vi "PruebaCalibration.vi"() -> ()   [LabVIEW 2014, in "MSX-E3701_dll.lvlib"]
uses:
  MSX-E3701_dll.lvlib
  E:/Repositorio Magnis/INF002/v0/Modules/HAL/Drivers/Sync/ADDI-DATA MSX-E3701/API/MX370x.dll
  MX370x.dll
  Typedef/Connection Data.ctl
  E:/Repositorio Magnis/INF002/v0/Modules/HAL/Drivers/Sync/ADDI-DATA MSX-E3701/API/MXCommon.dll
  MXCommon.dll
panel:
  in  "Connection Data In":T1
  out "ulValue":u64
  out "TransducerGetNbrOfType":i32
  in  "stop":bool
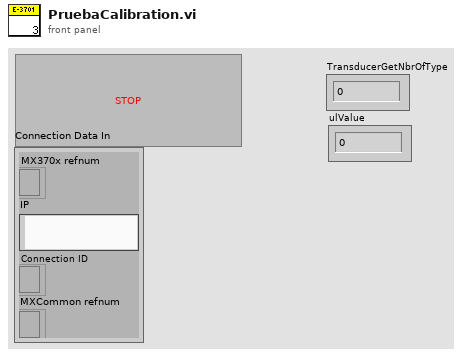
[diagram p1: front panel]
types:
  T1 = typedef "MSX-E3701_dll.lvlib/Connection Data.ctl" = cluster{"MX370x refnum":refnum<k24>, "IP":string, "Connection ID ":refnum<k5>, "MXCommon refnum":refnum<k24>}
  T2 = typedef "MSX-E3701_dll.lvlib/Calibration Data.ctl" = cluster{"Calibration status":string, "Name":string, "Index":u64, "Range":dbl, "Sensibility":dbl, "Veff":dbl, "Frequency":u64, "Impedance":u64, "Type":string, "Calibration Channel":u64}[]
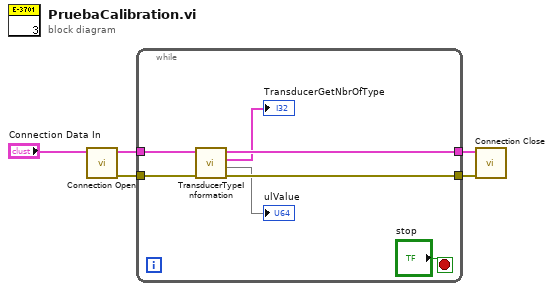
[diagram p0: block diagram]
diagram:
  n1 = call "Connection Open.vi"("Connection Data In"="Connection Data In") -> ("Error Out"=w3:errorcluster, "Connection Data Out"=w5:T1)  [unwired: 9 in]
  n2 = while {
    tunnel: w5 -> [w12]
    tunnel: [w11] -> w4
    tunnel: w3 -> [w10]
    tunnel: [w9] -> w2
    stop <- "stop" stop-if-true
    n3 = call "TransducerTypeInformation.vi"("error in (no error)"=w10, "Connection Data In"=w12) -> ("error out"=w9:errorcluster, 1:→"ulValue", "Cluster Calibration"=→"TransducerGetNbrOfType":T2, "Connection Data Out"=w11:T1)  [unwired: 6 in]
  }
  n4 = call "Connection Close.vi"("error in (no error)"=w2, "Connection Data In"=w4) -> ()  [unwired: 8 in, 2 out]
